vi "Get Temperature.vi"(6 "Channel":i32, 8 "error in (no error)":errorcluster, 11 "Instrument.Cryostat in":refnum<class "Instrument.Cryostat.lvclass">) -> (0 "error out":errorcluster, 1 "Status":string, 2 "Temperature (K)":dbl, 3 "Instrument.Cryostat out":refnum<class "Instrument.Cryostat.lvclass">, 4 "Finished?":bool)   [LabVIEW 2019, in "Instrument.Cryostat.lvclass"]
uses:
  Instrument.Cryostat.lvclass
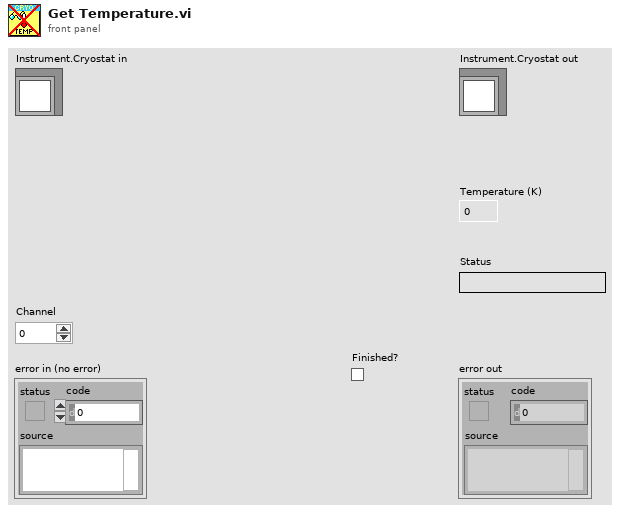
[diagram p1: front panel]
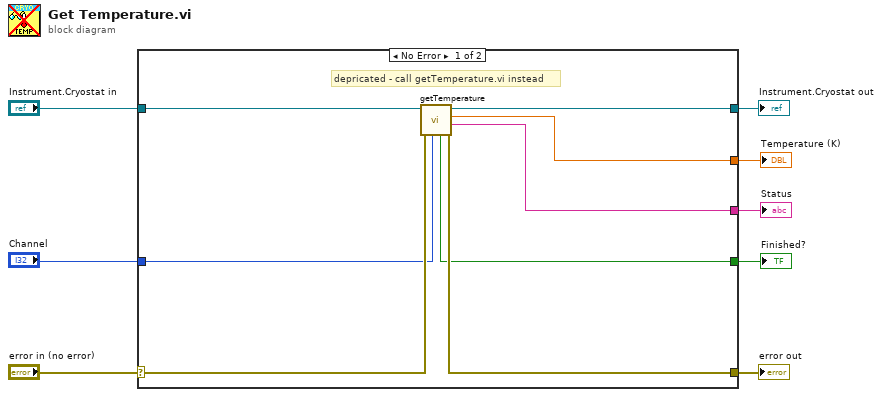
[diagram p0: block diagram]
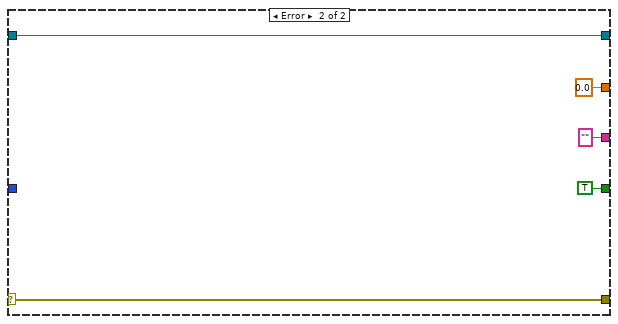
[diagram p2: hidden frame]
diagram:
  n1 = case shown="No Error" "error in (no error)" {
    selector: "error in (no error)" -> [w14 w21]
    tunnel: [w13 w21] -> w7
    tunnel: [w15 w20] -> w5
    tunnel: "Instrument.Cryostat in" -> [w16 w20]
    tunnel: "Channel" -> [w12 _]
    tunnel: [w11 TRUE ("Finished?")] -> w3
    tunnel: [w10 "" ("Status")] -> w2
    tunnel: [w9 0.0 ("Temperature (K)")] -> w1
    frame No Error {
      # "depricated - call getTemperature.vi instead"
      n2 = call-dynamic "getTemperature.vi"("Channel"=w12, "error in (no error)"=w14, "Instrument.Cryostat in"=w16) -> ("error out"=w13:errorcluster, "Status"=w10:string, "Temperature (K)"=w9:dbl, "Instrument.Cryostat out"=w15:refnum<class "Instrument.Cryostat.lvclass">, "Finished?"=w11:bool)  [unwired: 4 in]
    }
    frame Error {
    }
  }
  "error out" <- w7
  "Instrument.Cryostat out" <- w5
  "Temperature (K)" <- w1
  "Status" <- w2
  "Finished?" <- w3
